vi "_builtins_wire_error_structure.vi"(8 "error in (no error)":errorcluster, 11 "VI Refnum in":refnum<vi>) -> (0 "error out":errorcluster, 3 "VI Refnum out":refnum<vi>)   [LabVIEW 2019, in "Script.lvlib"]
doc: "Wires the error in and error out terminals of the selected case structure. If the case structure selector is already wired, this does nothing.\n\nCreated by: Ryan Pacini"
uses:
  Script.lvlib
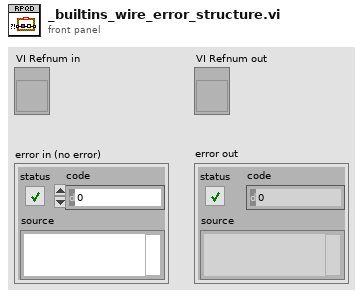
[diagram p1: front panel]
types:
  T1 = cluster{"in_tun":refnum<vi>, "in_term":refnum<vi>, "out_tun":refnum<vi>}
  T2 = typedef "LVPositionTypeDef.ctl" = cluster{"Left":i32, "Top":i32}
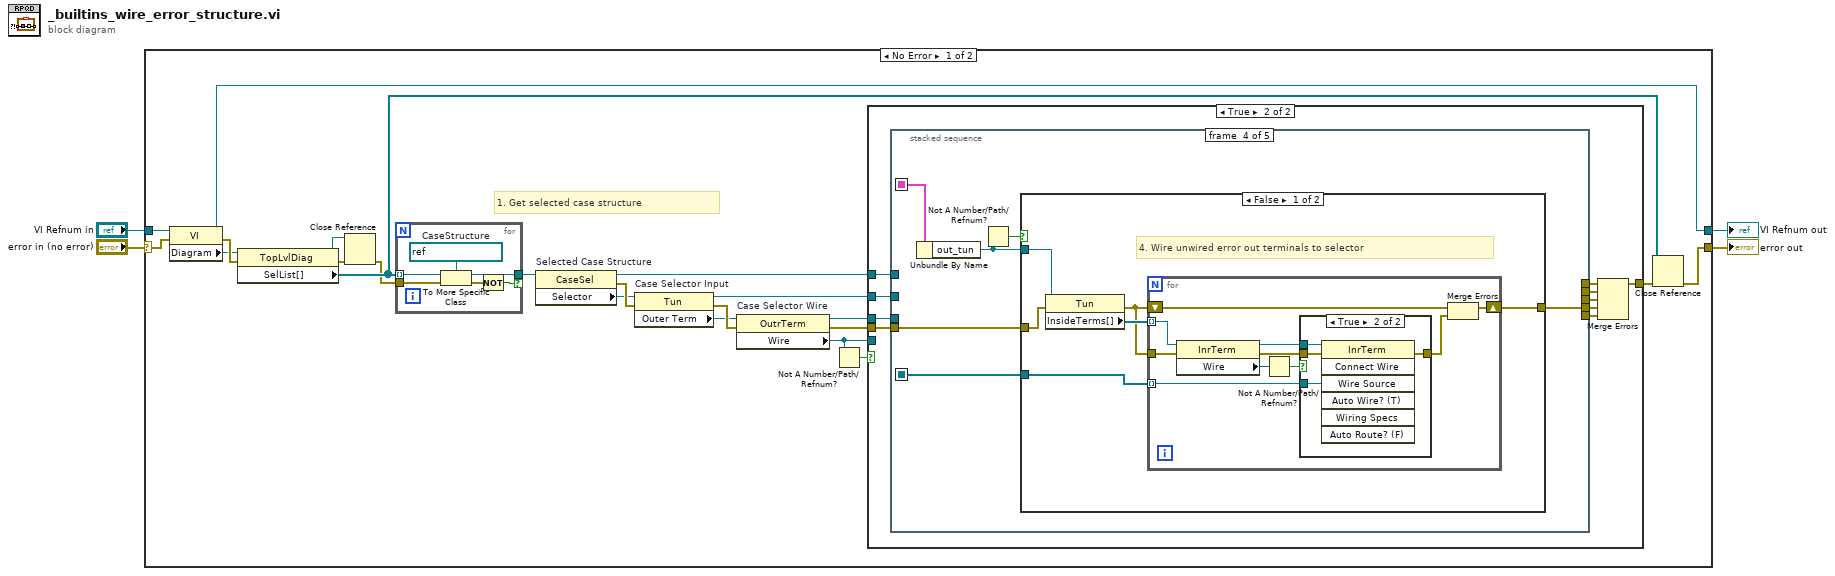
[diagram p0: block diagram]
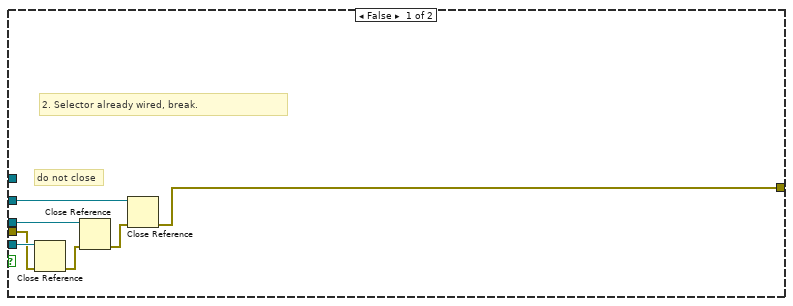
[diagram p2: hidden frame]
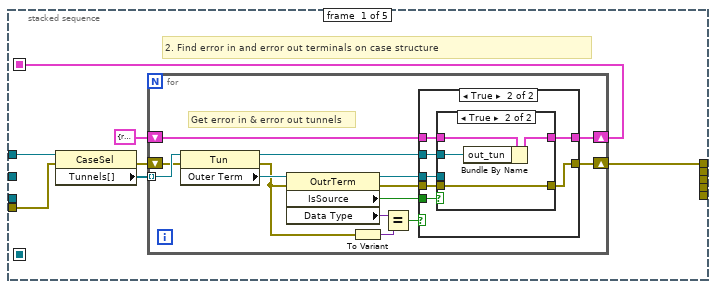
[diagram p3: hidden frame]
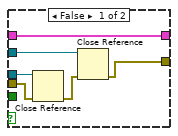
[diagram p4: hidden frame]
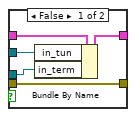
[diagram p5: hidden frame]
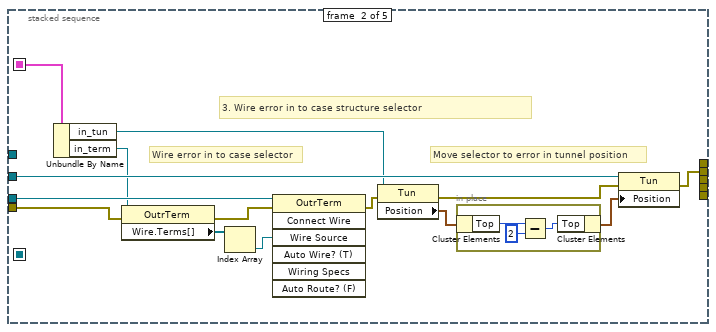
[diagram p6: hidden frame]
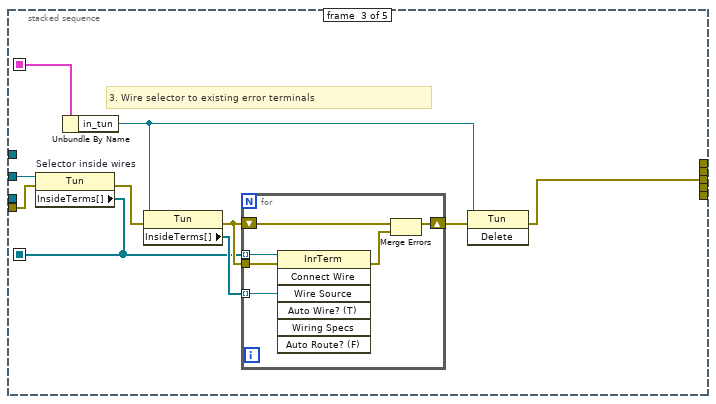
[diagram p7: hidden frame]
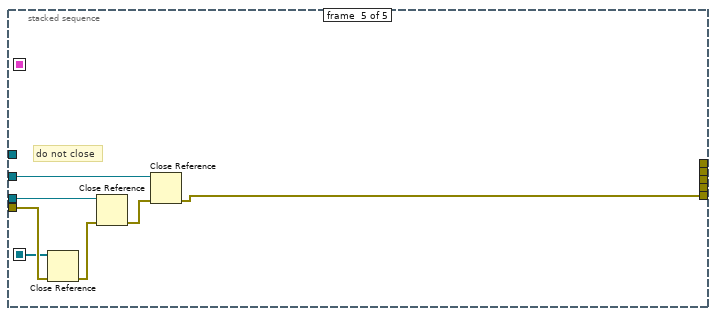
[diagram p10: hidden frame]
diagram:
  n1 = case shown="No Error" "error in (no error)" {
    selector: "error in (no error)" -> [w24 w161]
    tunnel: [w26 w162] -> w4
    tunnel: "VI Refnum in" -> [w25 w162]
    tunnel: [w5 w161] -> w1
    frame No Error {
      # "1. Get selected case structure"
      n2 = property class="VI"(reference=w25, error in=w24) -> (reference out=w26:refnum<vi>, error out=w10:errorcluster, "Diagram"=w6:refnum<vi>)
      n3 = property class="TopLvlDiag"(reference=w6, error in=w10) -> (reference out=w8:refnum<vi>, error out=w9:errorcluster, "SelList[]"=w11:refnum<vi>[])
      n4 = Close Reference(reference=w8, error in (no error)=w9) -> (error out=w7:errorcluster)
      n5 = for {
        tunnel: w11 -> [w159] mode=indexing
        tunnel: w7 -> [w160]
        tunnel: [w157] -> w12 if=w155
        w158 = refnum<vi> refnum  # CaseStructure
        n6 = To More Specific Class(target class=w158, reference=w159, error in=w160) -> (specific class reference=w157:refnum<vi>, error out=w156:errorcluster)
        n7 = Not(x=w156) -> (.not. x?=w155:bool)
      }
      n8 = property on="Selected Case Structure" class="CaseSel"(reference=w12) -> (reference out=w20:refnum<vi>, error out=w16:errorcluster, "Selector"=w13:refnum<vi>)  [unwired: 1 in]
      n9 = property on="Case Selector Input" class="Tun"(reference=w13, error in=w16) -> (reference out=w21:refnum<vi>, error out=w15:errorcluster, "Outer Term"=w14:refnum<vi>)
      n10 = property on="Case Selector Wire" class="OutrTerm"(reference=w14, error in=w15) -> (reference out=w22:refnum<vi>, error out=w19:errorcluster, "Wire"=w17:refnum<vi>)
      n11 = Not A Number/Path/Refnum?(number/path/refnum=w17) -> (NaN/Path/Refnum?=w18:bool)
      n12 = case shown="True" w18 {
        tunnel: w17 -> [w32 _]
        tunnel: w19 -> [w31 w42]
        tunnel: w20 -> [_ w43]
        tunnel: w21 -> [w33 w39]
        tunnel: w22 -> [w30 w38]
        tunnel: [w27 w40] -> w23
        frame False {
          # "2. Selector already wired, break."
          # "do not close"
          n13 = Close Reference(reference=w32, error in (no error)=w31) -> (error out=w29:errorcluster)
          n14 = Close Reference(reference=w30, error in (no error)=w29) -> (error out=w28:errorcluster)
          n15 = Close Reference(reference=w33, error in (no error)=w28) -> (error out=w27:errorcluster)
        }
        frame True {
          n16 = stacked-sequence {
            seq-local: [w45 _ _ _ _] -> [_ w100 w112 w124 _]
            seq-local: [_ _ w104 _ _] -> [_ _ _ w122 w148]
            tunnel: w43 -> [w47 _ _ _ _]
            tunnel: w42 -> [w46 w88 w107 w125 w154]
            tunnel: [w44 _ _ _ _] -> w41
            tunnel: w39 -> [_ w92 w105 _ w151]
            tunnel: w38 -> [_ w90 _ _ w153]
            tunnel: [_ w87 _ _ _] -> w37
            tunnel: [_ _ w108 _ _] -> w36
            tunnel: [_ _ _ w123 _] -> w35
            tunnel: [_ _ _ _ w149] -> w34
            frame #0 {
              # "2. Find error in and error out terminals on case structure"
              n17 = property class="CaseSel"(reference=w47, error in=w46) -> (error out=w49:errorcluster, "Tunnels[]"=w50:refnum<vi>[])  [unwired: 1 out]
              n18 = for {
                tunnel: w50 -> [w64] mode=indexing
                shift-right: [w55] -> w44
                shift-left: w49 -> [w63]
                shift-right: [w52] -> w45
                shift-left: T1 {"in_tun"=refnum, "in_term"=refnum, "out_tun"=refnum} ("ref") -> [w53]
                # "Get error in & error out tunnels"
                n19 = property class="Tun"(reference=w64, error in=w63) -> (reference out=w57:refnum<vi>, error out=w59:errorcluster, "Outer Term"=w62:refnum<vi>)
                n20 = property class="OutrTerm"(reference=w62, error in=w59) -> (reference out=w56:refnum<vi>, error out=w54:errorcluster, "IsSource"=w51:bool, "Data Type"=w61:variant)
                n21 = To Variant(anything=w59) -> (Variant=w60:variant)
                n22 = Equal?(x=w61, y=w60) -> (x = y?=w58:bool)
                n23 = case shown="True" w58 {
                  tunnel: w57 -> [w66 w76]
                  tunnel: w56 -> [w68 w75]
                  tunnel: [w67 w74] -> w55
                  tunnel: w54 -> [w70 w73]
                  tunnel: w51 -> [_ w77]
                  tunnel: w53 -> [w65 w72]
                  tunnel: [w65 w71] -> w52
                  frame False {
                    n24 = Close Reference(reference=w68, error in (no error)=w70) -> (error out=w69:errorcluster)
                    n25 = Close Reference(reference=w66, error in (no error)=w69) -> (error out=w67:errorcluster)
                  }
                  frame True {
                    n26 = case shown="True" w77 {
                      tunnel: w76 -> [w80 w85]
                      tunnel: w75 -> [w79 _]
                      tunnel: [w82 w86] -> w74
                      tunnel: w73 -> [w82 w86]
                      tunnel: w72 -> [w81 w84]
                      tunnel: [w78 w83] -> w71
                      frame False {
                        n27 = Bundle By Name(cluster=w81, "in_tun"=w80, "in_term"=w79) -> (w78:T1)
                      }
                      frame True {
                        n28 = Bundle By Name(cluster=w84, "out_tun"=w85) -> (w83:T1)
                      }
                    }
                  }
                }
              }
            }
            frame #1 {
              # "3. Wire error in to case structure selector"
              # "Move selector to error in tunnel position"
              # "Wire error in to case selector"
              n29 = Unbundle By Name(w100) -> ("in_tun"=w91:refnum<vi>, "in_term"=w89:refnum<vi>)
              n30 = property class="OutrTerm"(reference=w89, error in=w88) -> (error out=w95:errorcluster, "Wire.Terms[]"=w97:refnum<vi>[])  [unwired: 1 out]
              n31 = Index Array(array=w97) -> (element=w96:refnum<vi>)  [unwired: 1 in]
              n32 = invoke class="OutrTerm" method="Connect Wire"(reference=w90, error in=w95, "Wire Source"=w96) -> (error out=w99:errorcluster)  [unwired: 4 in, 6 out]
              n33 = property class="Tun"(reference=w91, error in=w99) -> (error out=w98:errorcluster, "Position"=w94:T2)  [unwired: 1 out]
              n34 = in-place {
                n35 = in-place-cluster #1(w94) -> ("Top"=w103:i32)
                n36 = Subtract(x=w103, y=2 ("x")) -> (x-y=w102:i32)
                n37 = in-place-cluster #1("Top"=w102) -> (w93:T2)
              }
              n38 = property class="Tun"(reference=w92, error in=w98, "Position"=w93) -> (error out=w87:errorcluster)  [unwired: 1 out]
            }
            frame #2 {
              # "3. Wire selector to existing error terminals"
              n39 = property on="Selector inside wires" class="Tun"(reference=w105, error in=w107) -> (error out=w106:errorcluster, "InsideTerms[]"=w104:refnum<vi>[])  [unwired: 1 out]
              n40 = Unbundle By Name(w112) -> ("in_tun"=w111:refnum<vi>)
              n41 = property class="Tun"(reference=w111, error in=w106) -> (error out=w110:errorcluster, "InsideTerms[]"=w113:refnum<vi>[])  [unwired: 1 out]
              n42 = for {
                tunnel: w110 -> [w119]
                tunnel: w104 -> [w117] mode=indexing
                tunnel: w113 -> [w116] mode=indexing
                shift-right: [w115] -> w109
                shift-left: w110 -> [w114]
                n43 = invoke class="InrTerm" method="Connect Wire"(reference=w117, error in=w119, "Wire Source"=w116) -> (error out=w118:errorcluster)  [unwired: 4 in, 6 out]
                n44 = Merge Errors(w114, w118) -> (w115:errorcluster)
              }
              n45 = invoke class="Tun" method="Delete"(reference=w111, error in=w109) -> (error out=w108:errorcluster)  [unwired: 1 in, 2 out]
            }
            frame #3 {
              n46 = Unbundle By Name(w124) -> ("out_tun"=w121:refnum<vi>)
              n47 = Not A Number/Path/Refnum?(number/path/refnum=w121) -> (NaN/Path/Refnum?=w120:bool)
              n48 = case shown="False" w120 {
                tunnel: w125 -> [w130 w147]
                tunnel: w121 -> [w129 _]
                tunnel: [w127 w147] -> w123
                tunnel: w122 -> [w126 _]
                frame False {
                  # "4. Wire unwired error out terminals to selector"
                  n49 = property class="Tun"(reference=w129, error in=w130) -> (error out=w128:errorcluster, "InsideTerms[]"=w131:refnum<vi>[])  [unwired: 1 out]
                  n50 = for {
                    tunnel: w131 -> [w140] mode=indexing
                    tunnel: w128 -> [w141]
                    tunnel: w126 -> [w135] mode=indexing
                    shift-right: [w133] -> w127
                    shift-left: w128 -> [w134]
                    n51 = property class="InrTerm"(reference=w140, error in=w141) -> (reference out=w136:refnum<vi>, error out=w137:errorcluster, "Wire"=w139:refnum<vi>)
                    n52 = Not A Number/Path/Refnum?(number/path/refnum=w139) -> (NaN/Path/Refnum?=w138:bool)
                    n53 = case shown="True" w138 {
                      tunnel: w137 -> [w142 w146]
                      tunnel: w136 -> [_ w145]
                      tunnel: w135 -> [_ w144]
                      tunnel: [w142 w143] -> w132
                      frame False {
                      }
                      frame True {
                        n54 = invoke class="InrTerm" method="Connect Wire"(reference=w145, error in=w146, "Wire Source"=w144) -> (error out=w143:errorcluster)  [unwired: 4 in, 6 out]
                      }
                    }
                    n55 = Merge Errors(w134, w132) -> (w133:errorcluster)
                  }
                }
                frame True {
                }
              }
            }
            frame #4 {
              # "do not close"
              n56 = Close Reference(reference=w148, error in (no error)=w154) -> (error out=w152:errorcluster)
              n57 = Close Reference(reference=w153, error in (no error)=w152) -> (error out=w150:errorcluster)
              n58 = Close Reference(reference=w151, error in (no error)=w150) -> (error out=w149:errorcluster)
            }
          }
          n59 = Merge Errors(w41, w37, w36, w35, w34) -> (w40:errorcluster)
        }
      }
      n60 = Close Reference(reference=w11, error in (no error)=w23) -> (error out=w5:errorcluster)
    }
    frame Error {
    }
  }
  "VI Refnum out" <- w4
  "error out" <- w1
